vi "Generated Descriptors.vi"() -> (3 "Descriptor Strings":string[](array[string]))   [LabVIEW 2025, in "reflection_server.lvlib"]
uses:
  reflection_server.lvlib
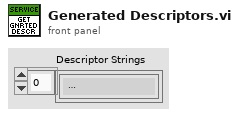
[diagram p1: front panel]
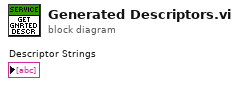
[diagram p0: block diagram]
diagram:
